vi "AutoHome.vi"(6 "Into Home Limit Is Pos":bool, 8 "Power In":dbl, 10 "Motor Ref":T4={"DeviceStatus"={"status"=FALSE, "code"=0, "source"=""}, "Type"=enum."PWM", "PWM"={"PWM Channel"=enum."Invalid", "DeadBand"={"Name"="", "maxPositivePwm"=0, "minPositivePwm"=0, "centerPwm"=0, "maxNegativePwm"=0, "minNegativePwm"=0, "angularRange"=0}}, "CAN"={"Device Number"=0, "SetOutput VI Ref"=variant, "GetOutput VI Ref"=variant, "Enable VI Ref"=variant, "Disable VI Ref"=variant, "Data"=variant}, "Invert"=FALSE, "DIO PWM"={"PWM \"Enable\" Channel"=enum."Invalid", "DIOChannel"=enum."Invalid", "PWM Rate"=0.0}}, 11 "Limit Switch Ref":T1={"DevStatus"={"status"=FALSE, "code"=0, "source"=""}, "DIO Channel"=enum."DIO 1", "CntIndex"=enum."Invalid", "Normally Closed"=FALSE}) -> (0 "Power Out":dbl, 3 "Done":bool)   [LabVIEW 2018]
uses:
  <vilib>/Rock Robotics/WPI/MotorControl/WPI_MotorControlDeviceRef.ctl
  <vilib>/Rock Robotics/WPI/MotorControl/WPI_MotorControlType.ctl
  <vilib>/Rock Robotics/SystemInterfaces/DIO/FPGA_DIOPWMChannel.ctl
  <vilib>/Rock Robotics/WPI/PWM/WPI_PWMDeadband.ctl
  <vilib>/Rock Robotics/SystemInterfaces/DIO/FPGA_DIOChannel.ctl
  <vilib>/Rock Robotics/WPI/Switch/WPI_SwitchDevRef.ctl
  <vilib>/Rock Robotics/SystemInterfaces/Counter/FPGA_CounterCtrSystemIndex.ctl
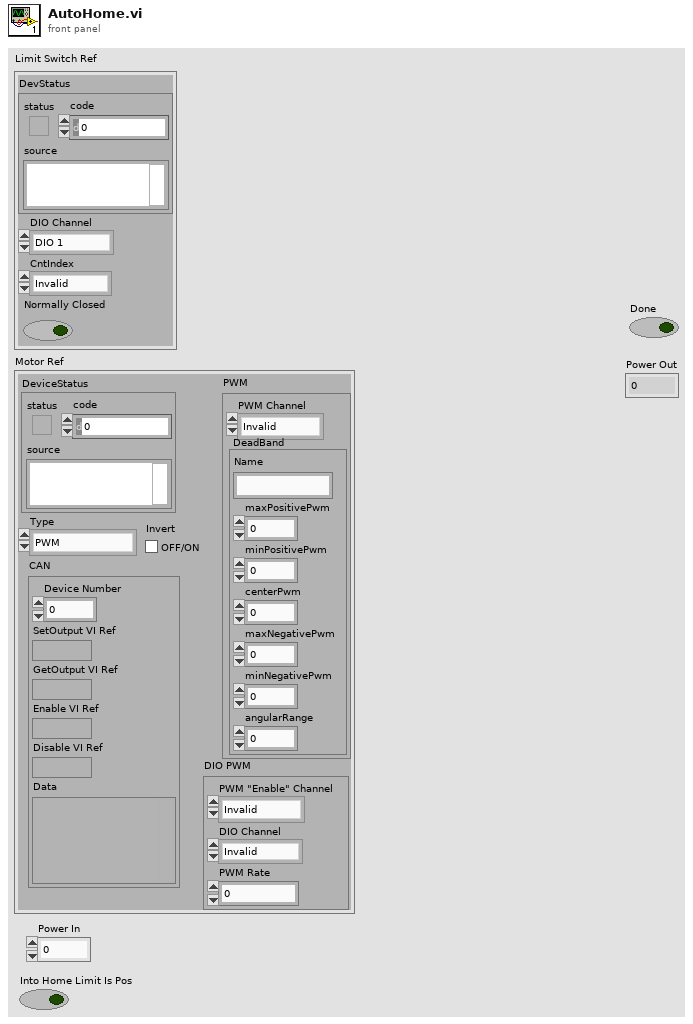
[diagram p1: front panel]
types:
  T1 = typedef "WPI_SwitchDevRef.ctl" = cluster{"DevStatus":errorcluster, "DIO Channel":T2, "CntIndex":T3, "Normally Closed":bool}
  T2 = typedef "FPGA_DIOChannel.ctl" = enum8{"DIO 0", "DIO 1", "DIO 2", "DIO 3", "DIO 4", "DIO 5", "DIO 6", "DIO 7", "DIO 8", "DIO 9", "DIO MXP 0", "DIO MXP 1", "DIO MXP 2", "DIO MXP 3", "DIO MXP 4", "DIO MXP 5", "DIO MXP 6", "DIO MXP 7", "DIO MXP 8", "DIO MXP 9", "DIO MXP 10", "DIO MXP 11", "DIO MXP 12", "DIO MXP 13", "DIO MXP 14", "DIO MXP 15", "SPI Port CS1", "SPI Port CS2", "SPI Port CS3", "SPI Port MISO", "SPI Port MOSI", "Invalid"}
  T3 = typedef "FPGA_CounterCtrSystemIndex.ctl" = enum8{"Ctr 0", "Ctr 1", "Ctr 2", "Ctr 3", "Ctr 4", "Ctr 5", "Ctr 6", "Ctr 7", "Invalid"}
  T4 = typedef "WPI_MotorControlDeviceRef.ctl" = cluster{"DeviceStatus":errorcluster, "Type":T5, "PWM":cluster{"PWM Channel":T6, "DeadBand":T7}, "CAN":cluster{"Device Number":u8, "SetOutput VI Ref":variant, "GetOutput VI Ref":variant, "Enable VI Ref":variant, "Disable VI Ref":variant, "Data":variant}, "Invert":bool, "DIO PWM":cluster{"PWM \"Enable\" Channel":T6, "DIOChannel":T2, "PWM Rate":dbl}}
  T5 = typedef "WPI_MotorControlType.ctl" = enum16{"PWM", "CAN", "DIO PWM"}
  T6 = typedef "FPGA_DIOPWMChannel.ctl" = enum8{"PWM 0", "PWM 1", "PWM 2", "PWM 3", "PWM 4", "PWM 5", "PWM 6", "PWM 7", "PWM 8", "PWM 9", "PWM MXP 0", "PWM MXP 1", "PWM MXP 2", "PWM MXP 3", "PWM MXP 4", "PWM MXP 5", "PWM MXP 6", "PWM MXP 7", "PWM MXP 8", "PWM MXP 9", "Invalid"}
  T7 = typedef "WPI_PWMDeadband.ctl" = cluster{"Name":string, "maxPositivePwm":i32, "minPositivePwm":i32, "centerPwm":i32, "maxNegativePwm":i32, "minNegativePwm":i32, "angularRange":u16}
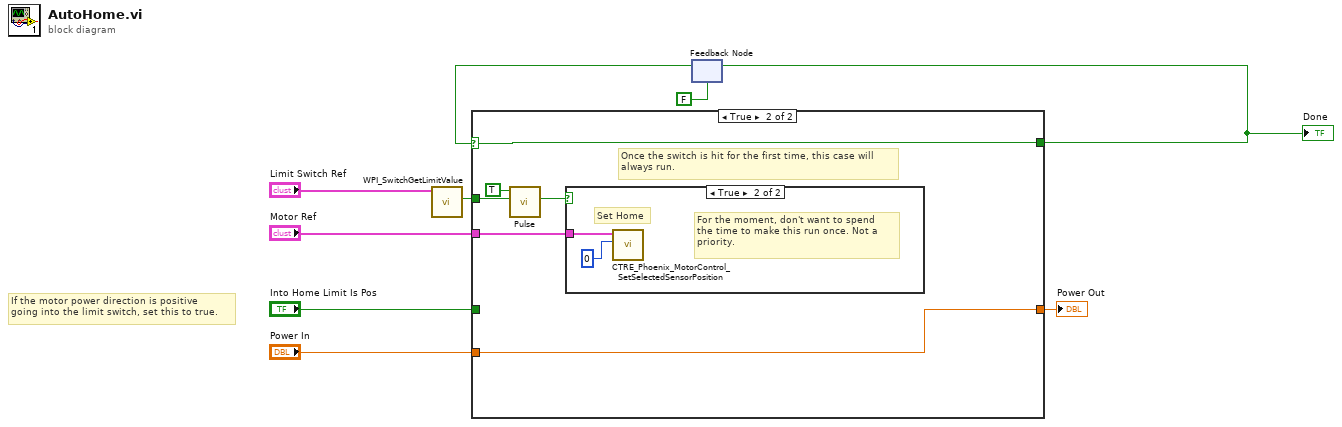
[diagram p0: block diagram]
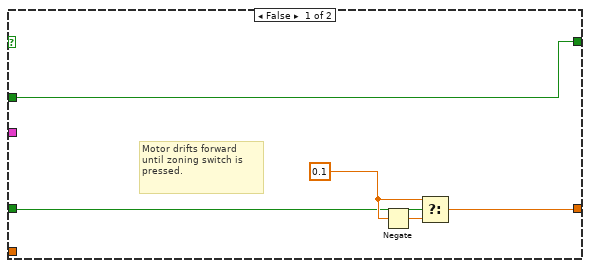
[diagram p2: hidden frame]
diagram:
  # "If the motor power direction is positive\ngoing into the limit switch, set this to true."
  n1 = call <vilib>:"WPI_SwitchGetLimitValue.vi"("SwitchDevRef"="Limit Switch Ref") -> ("Switch Pressed"=w9:bool)  [unwired: 8 in, 2 out]
  n2 = feedback #1(FALSE) -> (w7:bool)
  n3 = case shown="True" w7 {
    selector: w7 -> [_ w20]
    tunnel: [w14 w20] -> w1
    tunnel: w9 -> [w14 w17]
    tunnel: "Motor Ref" -> [_ w19]
    tunnel: [w10 w18] -> w6
    tunnel: "Into Home Limit Is Pos" -> [w11 _]
    tunnel: "Power In" -> [_ w18]
    frame False {
      w13 = 0.1 ("Output")
      # "Motor drifts forward until zoning switch is pressed."
      n4 = Negate(x=w13) -> (-x=w12:dbl)
      n5 = Select(t=w13, s=w11, f=w12) -> (s? t:f=w10:dbl)
    }
    frame True {
      # "Once the switch is hit for the first time, this case will \nalways run."
      n6 = call "Pulse.vi"("Input"=w17, "Rising Edge?"=TRUE) -> ("Output"=w16:bool)  [unwired: 9 in]
      n7 = case shown="True" w16 {
        tunnel: w19 -> [_ w21]
        frame False {
          # "Do \nNothing"
        }
        frame True {
          # "For the moment, don't want to spend \nthe time to make this run once. Not a\npriority."
          # "Set Home"
          n8 = call <vilib>:"CTRE_Phoenix_MotorControl_SetSelectedSensorPosition.vi"("New Sensor Position"=0, "PhoenixMotorControlDevRef"=w21) -> ()  [unwired: 8 in, 2 out]
        }
      }
    }
  }
  "Power Out" <- w6
  "Done" <- w1
  n9 = feedback-in #1(w1) -> ()
